vi "Win32-Hide Window.vi"(8 "error in (no error)":errorcluster, 11 "hWnd":i32) -> (0 "error out":errorcluster)   [LabVIEW 2015]
doc: "Uses Windows API to force panel to stay on top of all other windows."
uses:
  user32.dll
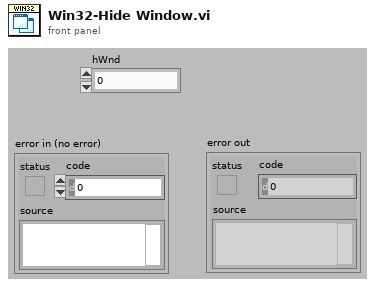
[diagram p1: front panel]
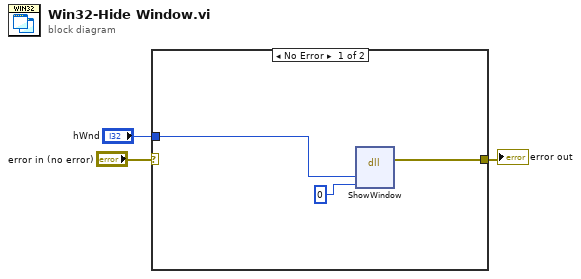
[diagram p0: block diagram]
diagram:
  n1 = case shown="No Error" "error in (no error)" {
    selector: "error in (no error)" -> [_ w7]
    tunnel: [w6 w7] -> w3
    tunnel: "hWnd" -> [w5 _]
    frame No Error {
      n2 = dll-call lib="user32.dll" fn="ShowWindow"("hWnd"=w5, "nCmdShow"=0 ("hWndInsertAfter")) -> (error out=w6:errorcluster)  [unwired: 5 in, 2 out]
    }
    frame Error {
    }
  }
  "error out" <- w3
